vi "Renishaw-XL80_GetOpticsFactor.vi"(8 "error in (no error)":errorcluster, 11 "Renishaw-XL80_EMU in":refnum<class "Renishaw-XL80_EMU.lvclass">) -> (0 "error out":errorcluster, 2 "OpticsFactor":dbl, 3 "Renishaw-XL80_EMU out":refnum<class "Renishaw-XL80_EMU.lvclass">)   [LabVIEW 2024, in "Renishaw-XL80_EMU.lvclass"]
doc: "Reading this property retrieves the current optics factor.\n\nDefinition\nHRESULTget_OpticsFactor( [out, retval] double* pVal);\nParameters\npVal\nA variable that will be set to the current optics factor.\n\nComments\nReading this property will always retrieve the current optics factor.\n\nThe property will normally return an HRESULT of S_OK. However, it will return E_POINTER if the client supplies a null pointer for pVal."
uses:
  Renishaw-XL80_EMU.lvclass
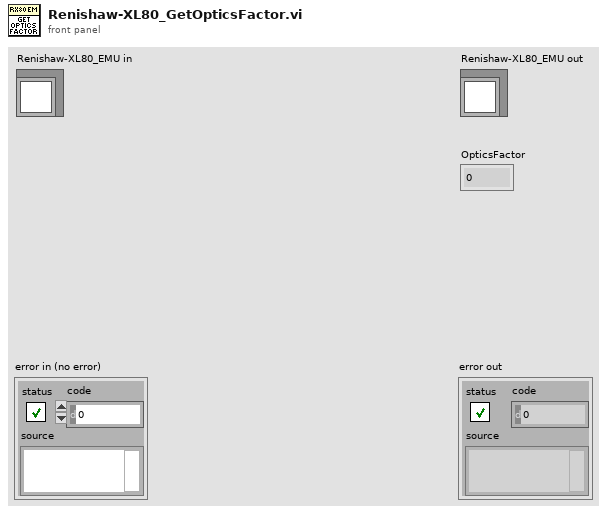
[diagram p1: front panel]
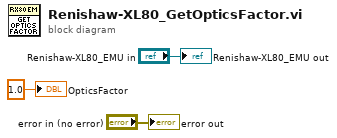
[diagram p0: block diagram]
diagram:
  "error out" <- "error in (no error)"
  "Renishaw-XL80_EMU out" <- "Renishaw-XL80_EMU in"
  "OpticsFactor" <- 1.0 ("OpticsFactor")
